vi "max_peaks.vi"(1 "FFT in":dbl[][](array[numeric])) -> (0 "peak indices":i32[](array[numeric]))   [LabVIEW 2009]
uses:
  <vilib>/Analysis/NI_AALBase.lvlib
panel:
  out "peaks":dbl[](array[numeric])
  out "XY Graph":cluster{"FFT in":dbl[], "FFT in":dbl[]}(graph)
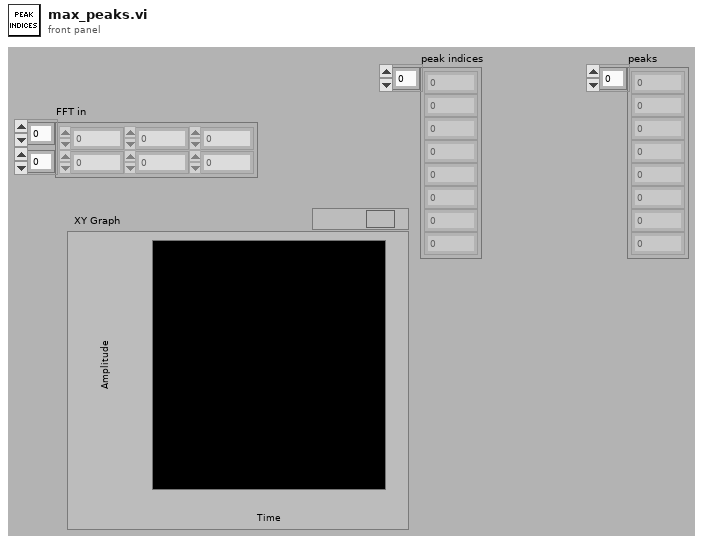
[diagram p1: front panel]
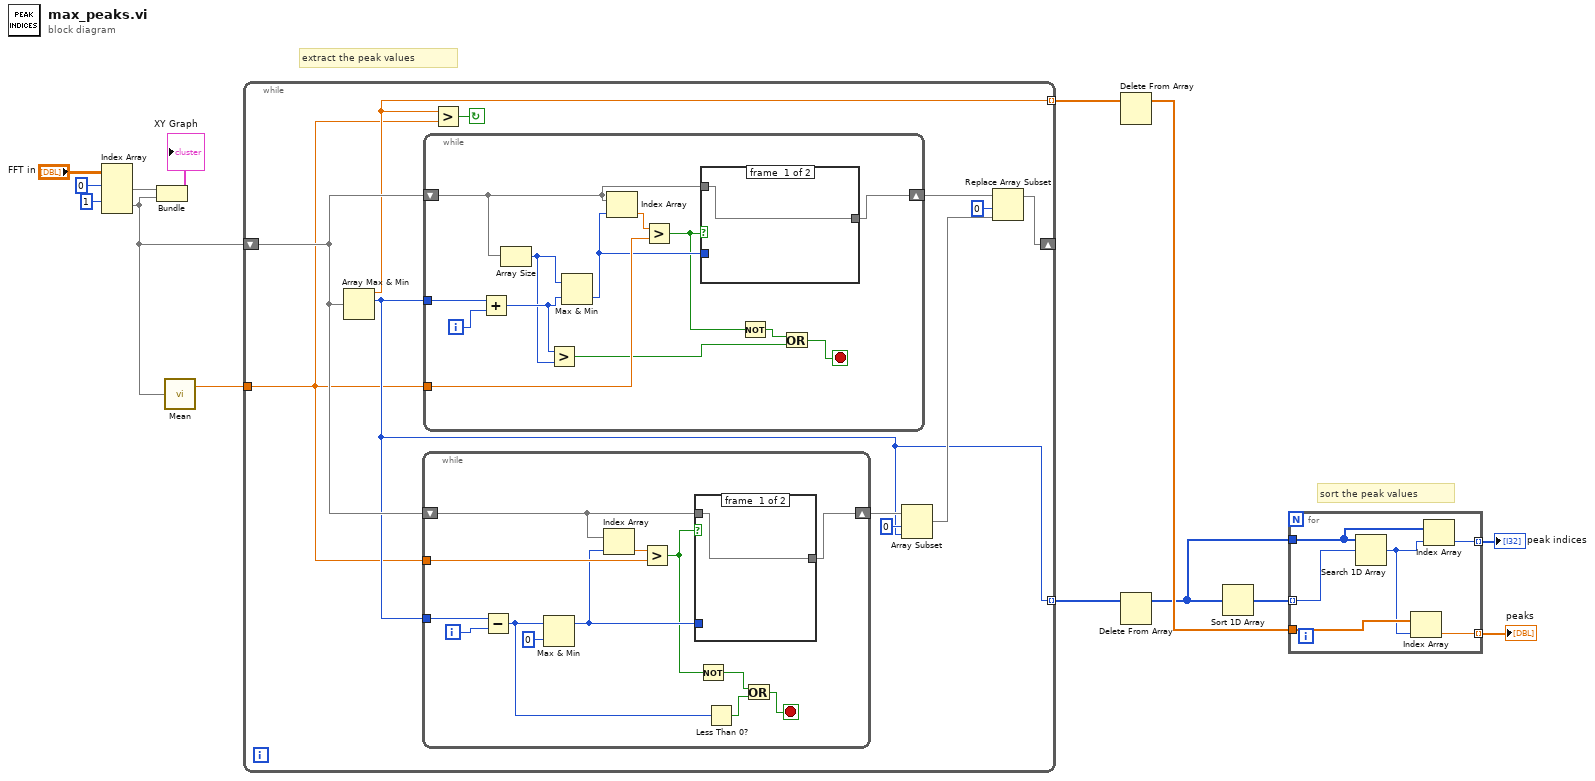
[diagram p0: block diagram]
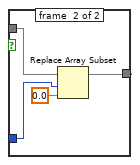
[diagram p2: hidden frame]
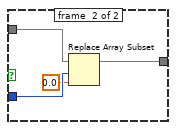
[diagram p3: hidden frame]
diagram:
  # "extract the peak values"
  # "sort the peak values"
  n1 = Index Array(array="FFT in", index (row) #1=0 ("index (row)"), index (row) #2=1 ("index (row)")) -> (element #1=w10:dbl[], element #2=w9:dbl[])  [unwired: 2 in]
  n2 = Bundle("FFT in"=w10, "FFT in"=w9) -> (→"XY Graph":cluster{"FFT in":dbl[], "FFT in":dbl[]})  [unwired: 1 in]
  n3 = call <vilib>:"Mean.vi"("X"=w9) -> ("mean"=w12:dbl)  [unwired: 1 out]
  n4 = while {
    tunnel: w12 -> [w15]
    shift-right: [w19] -> _
    shift-left: w9 -> [w25]
    tunnel: [w18] -> w5 mode=indexing
    tunnel: [w16] -> w3 mode=indexing
    stop <- w17 continue-if-true
    n5 = Array Max & Min(array=w25) -> (max value=w18:dbl, max index (indices)=w16:i32)  [unwired: 2 out]
    n6 = while {
      tunnel: w16 -> [w38]
      shift-right: [w34] -> w23
      shift-left: w25 -> [w32]
      tunnel: w15 -> [w36]
      i -> [w31]
      stop <- w28 stop-if-true
      n7 = Subtract(x=w38, y=w31) -> (x-y=w30:i32)
      n8 = Max & Min(x=w30, y=0) -> (max(x,y)=w35:i32)  [unwired: 1 out]
      n9 = Index Array(array=w32, index=w35) -> (element=w33:dbl)
      n10 = Greater?(x=w33, y=w36) -> (0:w27:bool)
      n11 = case shown="True" w27 {
        tunnel: w35 -> [_ w43]
        tunnel: [w39 w41] -> w34
        tunnel: w32 -> [w39 w40]
        frame #0 {
        }
        frame #1 {
          n12 = Replace Array Subset(array=w40, new element=0.0 ("new element/subarray"), index=w43) -> (w41:dbl[])
        }
      }
      n13 = Not(x=w27) -> (.not. x?=w26:bool)
      n14 = Less Than 0?(x=w30) -> (x < 0?=w29:bool)
      n15 = Or(x=w26, y=w29) -> (x .or. y?=w28:bool)
    }
    n16 = while {
      tunnel: w16 -> [w56]
      shift-right: [w50] -> w24
      shift-left: w25 -> [w52]
      tunnel: w15 -> [w53]
      i -> [w55]
      stop <- w47 stop-if-true
      n17 = Add(x=w56, y=w55) -> (x+y=w49:i32)
      n18 = Array Size(array=w52) -> (size(s)=w48:i32)
      n19 = Greater?(x=w49, y=w48) -> (0:w46:bool)
      n20 = Max & Min(x=w48, y=w49) -> (min(x,y)=w51:i32)  [unwired: 1 out]
      n21 = Index Array(array=w52, index=w51) -> (element=w54:dbl)
      n22 = Greater?(x=w54, y=w53) -> (0:w45:bool)
      n23 = case shown="True" w45 {
        tunnel: w52 -> [w57 w61]
        tunnel: w51 -> [_ w60]
        tunnel: [w57 w58] -> w50
        frame #0 {
        }
        frame #1 {
          n24 = Replace Array Subset(array=w61, new element=0.0 ("new element/subarray"), index=w60) -> (w58:dbl[])
        }
      }
      n25 = Not(x=w45) -> (.not. x?=w44:bool)
      n26 = Or(x=w44, y=w46) -> (x .or. y?=w47:bool)
    }
    n27 = Greater?(x=w18, y=w15) -> (0:w17:bool)
    n28 = Array Subset(array=w23, index=0, length=w16) -> (w21:dbl[])
    n29 = Replace Array Subset(array=w24, new element=w21, index=0) -> (w19:dbl[])
  }
  n30 = Delete From Array(array=w5) -> (array with subset deleted=w4:dbl[])  [unwired: 2 in, 1 out]
  n31 = Delete From Array(array=w3) -> (array with subset deleted=w2:i32[])  [unwired: 2 in, 1 out]
  n32 = Sort 1D Array(array=w2) -> (sorted array=w7:i32[])
  n33 = for {
    tunnel: w2 -> [w64]
    tunnel: w7 -> [w67] mode=indexing
    tunnel: w4 -> [w66]
    tunnel: [w65] -> w6 mode=indexing
    tunnel: [w62] -> w1 mode=indexing
    n34 = Search 1D Array(1D array=w64, element=w67) -> (index of element=w63:i32)  [unwired: 1 in]
    n35 = Index Array(array=w66, index=w63) -> (element=w65:dbl)
    n36 = Index Array(array=w64, index=w63) -> (element=w62:i32)
  }
  "peaks" <- w6
  "peak indices" <- w1
